vi "visualization_sub.vi"(10 "Latest?":bool, 11 "Instance":i32) -> (0 "ENC_VEL_Array":u16[](array[numeric]), 1 "ENC_POS_Array":i32[](array[numeric]), 2 "ADC_Array":dbl[](array[numeric]), 3 "Analog Data Cluster":T1, 4 "DIN":u16, 5 "dataToRead?":bool, 6 "Message Count":u32)   [LabVIEW 2022 SP3]
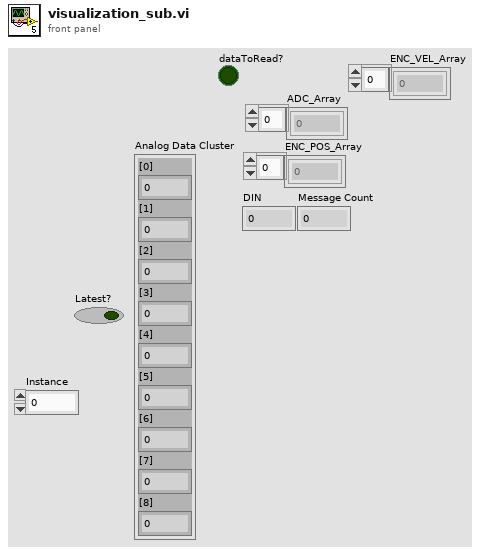
[diagram p1: front panel]
types:
  T1 = cluster{"[0]":dbl, "[1]":dbl, "[2]":dbl, "[3]":dbl, "[4]":dbl, "[5]":dbl, "[6]":dbl, "[7]":dbl, "[8]":dbl}
  T2 = cluster{"ADC_Array[0]":dbl, "ADC_Array[1]":dbl, "ADC_Array[2]":dbl, "ADC_Array[3]":dbl, "ADC_Array[4]":dbl, "ADC_Array[5]":dbl, "ADC_Array[6]":dbl, "ADC_Array[7]":dbl, "ADC_Array[8]":dbl}
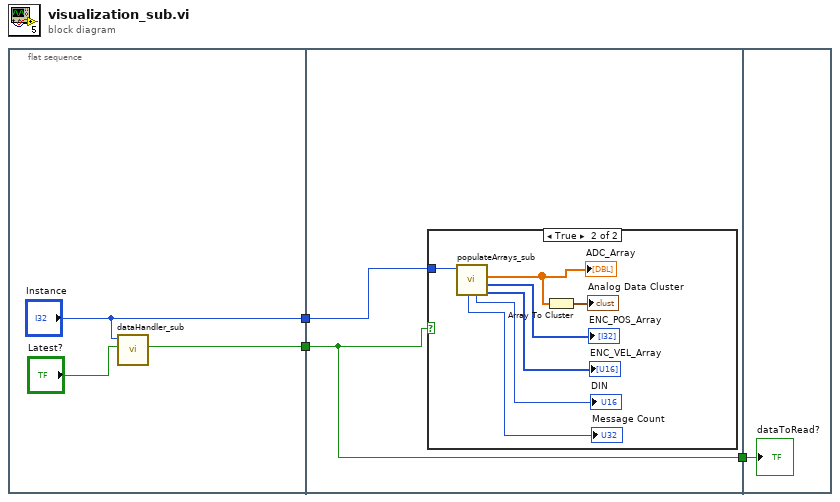
[diagram p0: block diagram]
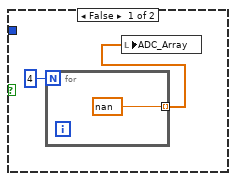
[diagram p2: hidden frame]
diagram:
  n1 = flat-sequence {
    tunnel: ["Instance"] -> w3
    tunnel: [w4] -> w2
    tunnel: w3 -> [w8]
    tunnel: w2 -> [w7]
    tunnel: [w7] -> w1
    tunnel: w1 -> [w19]
    frame #0 {
      n2 = call "dataHandler_sub.vi"("Instance"="Instance", "Latest?"="Latest?") -> ("dataToRead?"=w4:bool)  [unwired: 7 in, 1 out]
    }
    frame #1 {
      n3 = case shown="True" w7 {
        tunnel: w8 -> [_ w18]
        frame False {
          n4 = for {
            N: 4 -> [_]
            tunnel: [nan] -> w9 mode=indexing
          }
          n5 = local write "ADC_Array"(w9) -> ()
        }
        frame True {
          n6 = call "populateArrays_sub.vi"("Instance"=w18) -> ("ENC_VEL_Array"=→"ENC_VEL_Array":u16[], "ENC_POS_Array"=→"ENC_POS_Array":i32[], "ADC_Array"=w16:dbl[], "DIN"=→"DIN":u16, "Message Count"=→"Message Count":u32)  [unwired: 5 in, 1 out]
          "ADC_Array" <- w16
          n7 = Array To Cluster(array=w16) -> (cluster=→"Analog Data Cluster":T2)
        }
      }
    }
    frame #2 {
      "dataToRead?" <- w19
    }
  }
